vi "Read Pots.vi"() -> (0 "Pot Write Cluster":T1, 2 "Right Pot":dbl, 3 "Left Pot":dbl, 4 "Unzeroed Right Pot":dbl, 6 "Unzeroed Left Pot":dbl)   [LabVIEW 2015]
uses:
  Pot Data.ctl
  Robot Global Data.vi
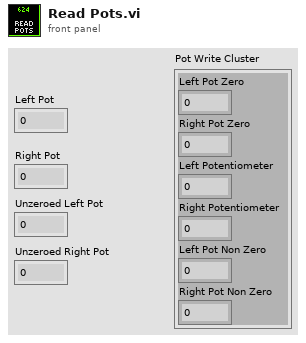
[diagram p1: front panel]
types:
  T1 = typedef "Pot Data.ctl" = cluster{"Left Pot Zero":sgl, "Right Pot Zero":sgl, "Left Potentiometer":sgl, "Right Potentiometer":sgl, "Left Pot Non Zero":sgl, "Right Pot Non Zero":sgl}
  T2 = typedef "Dashboard Control Data.ctl" = cluster{"Auton Loops":dbl, "Shooter Presets":T3, "Encoder Control":T5, "Intake Command Cluster ":cluster{"Intake Speed":dbl, "HP Load Speed":dbl, "Turn Out Speed":dbl, "Turn In Speed":dbl, "Unload Speed":dbl, "Right Pot 0":dbl, "Left Pot 0":dbl, "Right Pot Scale":dbl, "Left Pot Scale":dbl}}
  T3 = typedef "Shooter Presets.ctl" = cluster{"Batter Shot":T4, "Low Bar Curve Shot":T4, "Deep Middle Shot":T4, "Manual Shot":T4}
  T4 = typedef "Shot Presets.ctl" = cluster{"Left Wheel RPM":dbl, "Right Wheel RPM":dbl}
  T5 = typedef "Encoder Control.ctl" = cluster{"Right Tick Constat":dbl, "Left Tick Constant":dbl, "Reset?":bool, "Y Dist":cluster{"PID gains":cluster{"proportional gain (Kc)":dbl, "integral time (Ti, min)":dbl, "derivative time (Td<min)":dbl}}, "Y Stop Thresh":dbl, "Y Stop Speed":dbl}
  T6 = typedef "WPI_PotentiometerDevRef.ctl" = cluster{"DevStatus":errorcluster, "Analog Channel":T7, "Invert Output":bool}
  T7 = typedef "FPGA_AIChannel.ctl" = enum8{"AI 0", "AI 1", "AI 2", "AI 3", "AI MXP 0", "AI MXP 1", "AI MXP 2", "AI MXP 3", "Invalid"}
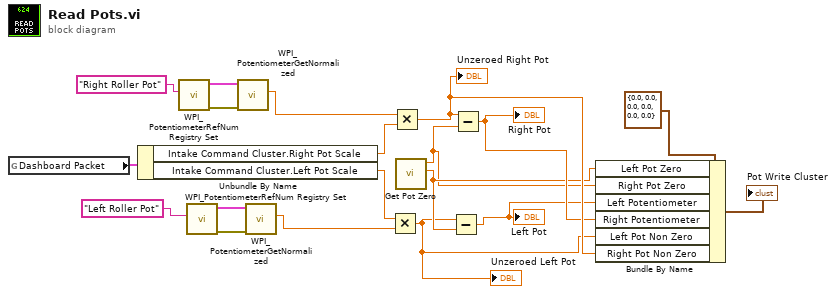
[diagram p0: block diagram]
diagram:
  n1 = global read "Robot Global Data.vi" "Dashboard Packet"() -> (w3:T2)
  n2 = Unbundle By Name(w3) -> ("Intake Command Cluster.Right Pot Scale"=w2:dbl, "Intake Command Cluster.Left Pot Scale"=w1:dbl)
  n3 = call <vilib>:"WPI_PotentiometerRefNum Registry Set.vi"("refnum name"="Right Roller Pot") -> ("error out"=w19:errorcluster, "PotDevRef"=w18:T6)  [unwired: 9 in]
  n4 = call <vilib>:"WPI_PotentiometerRefNum Registry Set.vi"("refnum name"="Left Roller Pot") -> ("error out"=w16:errorcluster, "PotDevRef"=w17:T6)  [unwired: 9 in]
  n5 = call <vilib>:"WPI_PotentiometerGetNormalized.vi"("error in"=w19, "PotDevRef"=w18) -> ("Normalized Value"=w13:dbl)  [unwired: 7 in, 2 out]
  n6 = call <vilib>:"WPI_PotentiometerGetNormalized.vi"("error in"=w16, "PotDevRef"=w17) -> ("Normalized Value"=w12:dbl)  [unwired: 7 in, 2 out]
  n7 = Multiply(x=w1, y=w12) -> (x*y=w4:dbl)
  "Unzeroed Left Pot" <- w4
  n8 = Multiply(x=w13, y=w2) -> (x*y=w9:dbl)
  "Unzeroed Right Pot" <- w9
  n9 = call "Get Pot Zero.vi"() -> ("Left Pot 0"=w7:dbl, "Right Pot 0"=w6:dbl)  [unwired: 10 in]
  n10 = Subtract(x=w4, y=w7) -> (x-y=w5:dbl)
  "Left Pot" <- w5
  n11 = Subtract(x=w9, y=w6) -> (x-y=w8:dbl)
  "Right Pot" <- w8
  n12 = Bundle By Name(cluster=T1 {"Left Pot Zero"=0.0, "Right Pot Zero"=0.0, "Left Potentiometer"=0.0, "Right Potentiometer"=0.0, "Left Pot Non Zero"=0.0, "Right Pot Non Zero"=0.0} ("Potentiometer Cluster"), "Left Pot Zero"=w7, "Right Pot Zero"=w6, "Left Potentiometer"=w5, "Right Potentiometer"=w8, "Left Pot Non Zero"=w4, "Right Pot Non Zero"=w9) -> (→"Pot Write Cluster":T1)
